vi "medie7.vi"(11 "Temperatura curenta":dbl) -> (3 "Numeric":dbl)   [LabVIEW 2014]
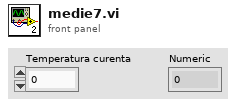
[diagram p1: front panel]
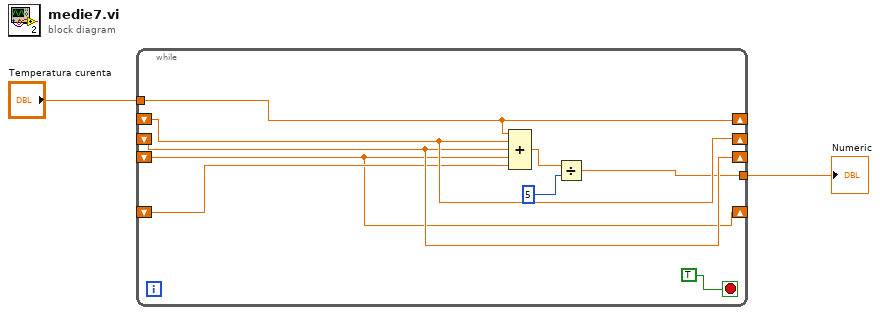
[diagram p0: block diagram]
diagram:
  n1 = while {
    shift-right: [w3] -> _
    shift-left: _ -> [w8]
    shift-right: [w8] -> _
    shift-left: _ -> [w7]
    shift-right: [w7] -> _
    shift-left: _ -> [w5]
    shift-right: [w5] -> _
    shift-left: _ -> [w6]
    tunnel: [w4] -> w1
    tunnel: "Temperatura curenta" -> [w3]
    stop <- TRUE stop-if-true
    n2 = Compound Arithmetic op=ADD(w3, w8, w7, w5, w6) -> (w11:dbl)
    n3 = Divide(x=w11, y=5 ("Numeric 2")) -> (x/y=w4:dbl)
  }
  "Numeric" <- w1
